vi "create_files.vi"(11 "project name":string) -> (1 "converter2":path, 2 "converter1":path, 3 "controller":path)   [LabVIEW 2019]
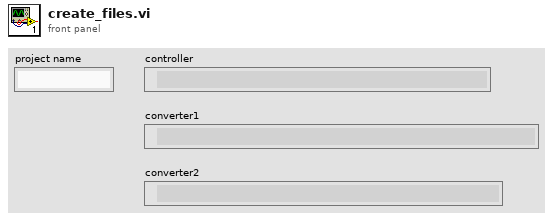
[diagram p1: front panel]
types:
  T1 = enum16{"open", "open or create", "create or replace", "create", "open (read only)"}
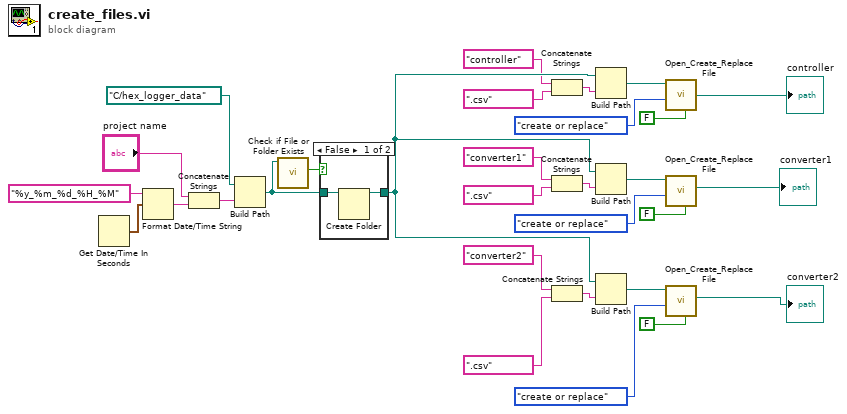
[diagram p0: block diagram]
diagram:
  n1 = Get Date/Time In Seconds() -> (seconds since 1Jan1904=w22:timestamp)
  n2 = Format Date/Time String(time format string (%c)="%y_%m_%d_%H_%M", seconds (now)=w22) -> (date/time string=w24:string)  [unwired: 1 in]
  n3 = Concatenate Strings("project name", w24) -> (w25:string)
  n4 = Build Path(base path=path "C:/hex_logger_data", name or relative path=w25) -> (appended path=w26:path)
  n5 = call <vilib>:"Check if File or Folder Exists.vi"("path"=w26) -> ("file or folder exists?"=w27:bool)  [unwired: 8 in, 2 out]
  n6 = case shown="False" w27 {
    tunnel: [w31 w33] -> w20
    tunnel: w26 -> [w32 w33]
    frame False {
      n7 = Create Folder(path (use dialog)=w32) -> (created path=w31:path)  [unwired: 2 in, 2 out]
    }
    frame True {
    }
  }
  n8 = Concatenate Strings("controller", ".csv") -> (w14:string)
  n9 = Concatenate Strings("converter1", ".csv") -> (w9:string)
  n10 = Concatenate Strings("converter2", ".csv") -> (w19:string)
  n11 = Build Path(base path=w20, name or relative path=w14) -> (appended path=w12:path)
  n12 = Build Path(base path=w20, name or relative path=w9) -> (appended path=w7:path)
  n13 = Build Path(base path=w20, name or relative path=w19) -> (appended path=w17:path)
  n14 = call <vilib>:"Open_Create_Replace File.vi"("advisory dialog? (display:T)"=FALSE, "function (open:0)"=T1."create or replace", "file path"=w12) -> ("new file path"=→"controller":path)  [unwired: 5 in, 3 out]
  n15 = call <vilib>:"Open_Create_Replace File.vi"("advisory dialog? (display:T)"=FALSE, "function (open:0)"=T1."create or replace", "file path"=w7) -> ("new file path"=→"converter1":path)  [unwired: 5 in, 3 out]
  n16 = call <vilib>:"Open_Create_Replace File.vi"("advisory dialog? (display:T)"=FALSE, "function (open:0)"=T1."create or replace", "file path"=w17) -> ("new file path"=→"converter2":path)  [unwired: 5 in, 3 out]
